vi "USB-2000 MultiAi.vi"() -> ()   [LabVIEW 2016]
uses:
  <vilib>/Analysis/baseanly.llb/Mean (DBL).vi
  <vilib>/Analysis/NI_AALBase.lvlib
panel:
  out "mean":dbl caption="均值" format="%0.5f"
  out "数值":i32
  in  "ChanMode":u8=1
  in  "Range":sgl=10.0
  out "error out":errorcluster caption="错误输出"
  in  "停止":bool
  out "波形图":cluster{dbl, dbl, sgl[][]}(graph)
  in  "读取通道选择":T1={"CH 0"=TRUE, "CH 1"=TRUE, "CH 2"=TRUE, "CH 3"=TRUE, "CH 4"=TRUE, "CH 5"=TRUE, "CH 6"=TRUE, "CH 7"=TRUE, "CH 8"=FALSE, "CH 9"=FALSE, "CH 10"=FALSE, "CH 11"=FALSE, "CH 12"=FALSE, "CH 13"=FALSE, "CH 14"=FALSE, "CH 15"=FALSE}
  in  "Num":u32=1000 caption="每通道读取点数"
  in  "SampleRate":u32=100000 caption="SampleRate (pts/s)"
  # "1：单端输入。\n0：差分输入。\n     选择差分输入时，只能勾选0,2,4...这样的偶数通道。"
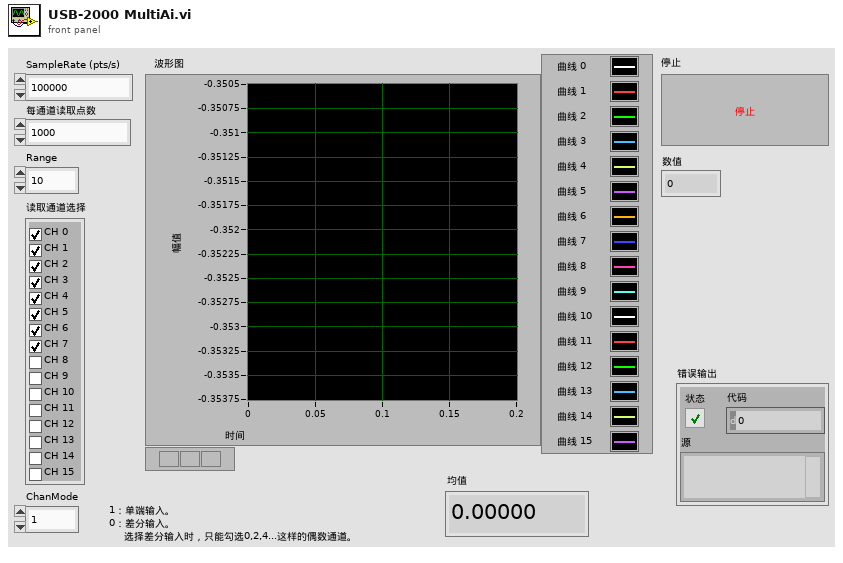
[diagram p1: front panel]
types:
  T1 = cluster{"CH 0":bool, "CH 1":bool, "CH 2":bool, "CH 3":bool, "CH 4":bool, "CH 5":bool, "CH 6":bool, "CH 7":bool, "CH 8":bool, "CH 9":bool, "CH 10":bool, "CH 11":bool, "CH 12":bool, "CH 13":bool, "CH 14":bool, "CH 15":bool}
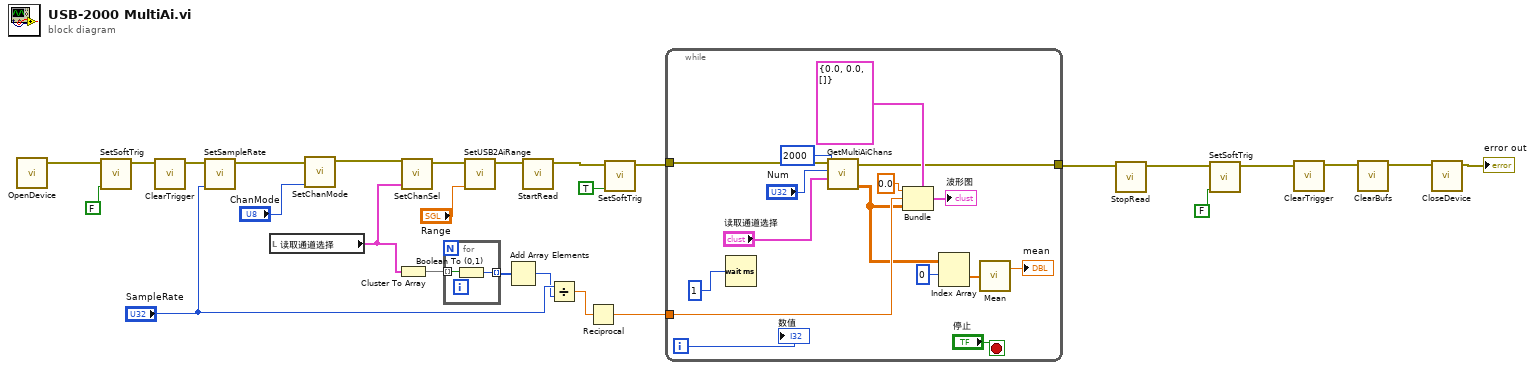
[diagram p0: block diagram]
diagram:
  n1 = call "OpenDevice.vi"() -> ("error out"=w24:errorcluster)  [unwired: 11 in]
  n2 = call "SetSoftTrig.vi"("SoftTrig"=FALSE, "error in"=w24) -> ("error out"=w7:errorcluster)  [unwired: 9 in]
  n3 = call "ClearTrigger.vi"("错误输入（无错误）"=w7) -> ("错误输出"=w9:errorcluster)  [unwired: 10 in]
  n4 = call "SetSampleRate.vi"("SampleRate"="SampleRate", "error in"=w9) -> ("error out"=w18:errorcluster)  [unwired: 9 in]
  n5 = local read "读取通道选择"() -> (w16:T1)
  n6 = call "SetChanMode.vi"("ChanMode"="ChanMode", "错误输入"=w18) -> ("错误输出"=w17:errorcluster)  [unwired: 9 in]
  n7 = Cluster To Array(cluster=w16) -> (array=w15:bool[])
  n8 = call "SetChanSel.vi"("读取通道选择"=w16, "错误输入"=w17) -> ("错误输出"=w19:errorcluster)  [unwired: 9 in]
  n9 = for {
    tunnel: w15 -> [w29] mode=indexing
    tunnel: [w28] -> w14 mode=indexing
    n10 = Boolean To (0,1)(Boolean=w29) -> (0, 1=w28:i16)
  }
  n11 = call "SetUSB2AiRange.vi"("Range"="Range", "error in"=w19) -> ("error out"=w4:errorcluster)  [unwired: 9 in]
  n12 = Add Array Elements(numeric array=w14) -> (sum=w12:i16)
  n13 = call "StartRead.vi"("error in"=w4) -> ("error out"=w5:errorcluster)  [unwired: 10 in]
  n14 = Divide(x="SampleRate", y=w12) -> (x/y=w11:dbl)
  n15 = Reciprocal(x=w11) -> (1/x=w21:dbl)
  n16 = call "SetSoftTrig.vi"("SoftTrig"=TRUE, "error in"=w5) -> ("error out"=w6:errorcluster)  [unwired: 9 in]
  n17 = while {
    tunnel: w6 -> [w45]
    tunnel: w21 -> [w38]
    tunnel: [w36] -> w1
    i -> [w35]
    stop <- "停止" stop-if-true
    n18 = Wait (ms)(milliseconds to wait=u32 1 ("等待时间（毫秒）")) -> ()  [unwired: 1 out]
    n19 = call "GetMultiAiChans.vi"("TimeOut (ms)"=2000, "ChansSel"="读取通道选择", "Num"="Num", "error in"=w45) -> ("Data"=w34:sgl[][], "error out"=w36:errorcluster)  [unwired: 6 in]
    n20 = Bundle(cluster=cluster{dbl, dbl, sgl[][]} {0.0, 0.0, []}, 0.0, w38, w34) -> (→"波形图":cluster{dbl, dbl, sgl[][]})
    n21 = Index Array(array=w34, index (row)=0 ("索引 (行)")) -> (element=w32:sgl[])  [unwired: 1 in]
    n22 = call-poly <vilib>:"Mean.vi"("X"=w32) -> ("mean"=→"mean":dbl)  [unwired: 1 out]
    "数值" <- w35
  }
  n23 = call "StopRead.vi"("error in"=w1) -> ("error out"=w2:errorcluster)  [unwired: 10 in]
  n24 = call "SetSoftTrig.vi"("SoftTrig"=FALSE, "error in"=w2) -> ("error out"=w3:errorcluster)  [unwired: 9 in]
  n25 = call "ClearTrigger.vi"("错误输入（无错误）"=w3) -> ("错误输出"=w25:errorcluster)  [unwired: 10 in]
  n26 = call "ClearBufs.vi"("error in"=w25) -> ("error out"=w27:errorcluster)  [unwired: 10 in]
  n27 = call "CloseDevice.vi"("error in"=w27) -> ("error out"=→"error out":errorcluster)  [unwired: 10 in]
